vi "For_Loop.vi"() -> ()   [LabVIEW 2022 SP3]
panel:
  out "Numeric 2":i32
  out "Waveform Chart":dbl(graph)
  out "Numeric":i32
  out "Boolean":bool
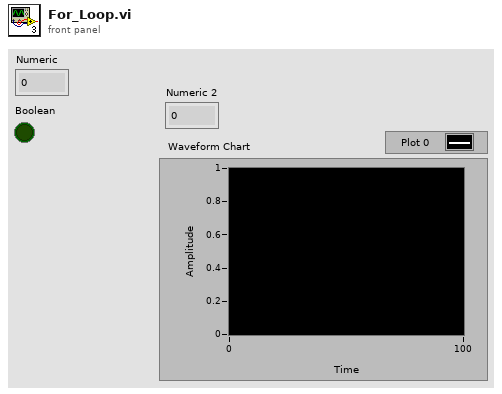
[diagram p1: front panel]
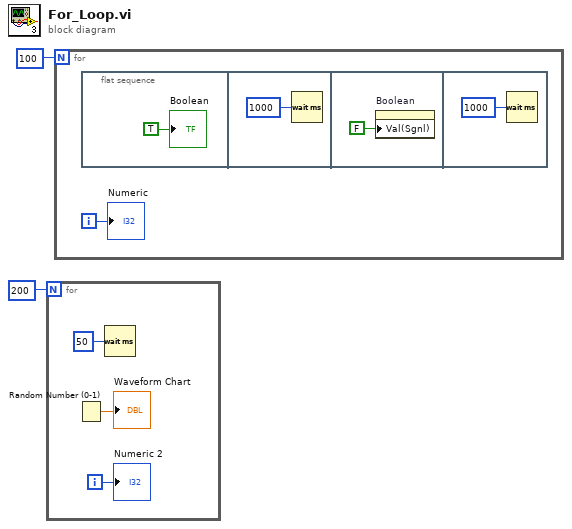
[diagram p0: block diagram]
diagram:
  n1 = for {
    N: 200 -> [_]
    i -> [w3]
    n2 = Random Number (0-1)() -> (number: 0 to 1=→"Waveform Chart":dbl)
    n3 = Wait (ms)(milliseconds to wait=u32 50 ("millisecond timer value")) -> ()  [unwired: 1 out]
    "Numeric 2" <- w3
  }
  n4 = for {
    N: 100 -> [_]
    i -> [w6]
    n5 = flat-sequence {
      frame #0 {
        "Boolean" <- TRUE ("Boolean")
      }
      frame #1 {
        n6 = Wait (ms)(milliseconds to wait=u32 1000 ("millisecond timer value")) -> ()  [unwired: 1 out]
      }
      frame #2 {
        n7 = property on="Boolean" class="Bool (strict)"("Val(Sgnl)"=FALSE ("Value (Signaling)")) -> ()  [unwired: 2 in, 2 out]
      }
      frame #3 {
        n8 = Wait (ms)(milliseconds to wait=u32 1000 ("millisecond timer value")) -> ()  [unwired: 1 out]
      }
    }
    "Numeric" <- w6
  }
